vi "Start.vi"(8 "error in (no error)":errorcluster, 11 "TDCManager":T1) -> (0 "error out":errorcluster, 1 "Added time":u64, 2 "Success?":bool=TRUE, 3 "TDCManager":T1)   [LabVIEW 2016, in "HPTDC Driver Library.lvlib"]
uses:
  HPTDC Driver Library.lvlib
  Typedefs/TDCManager.ctl
  C:/Users/CRT Controller/CRTC Labview Application/Source/HPTDC Driver Library Folder/Library files/hptdc_net4_3.7.0_x64.dll
  hptdc_net4_3.7.0_x64.dll
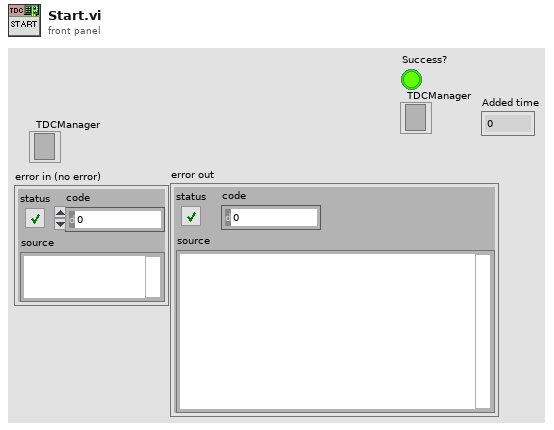
[diagram p1: front panel]
types:
  T1 = typedef "HPTDC Driver Library.lvlib/TDCManager.ctl" = refnum<k24>
  T2 = typedef "Semaphore RefNum" = refnum<k1>
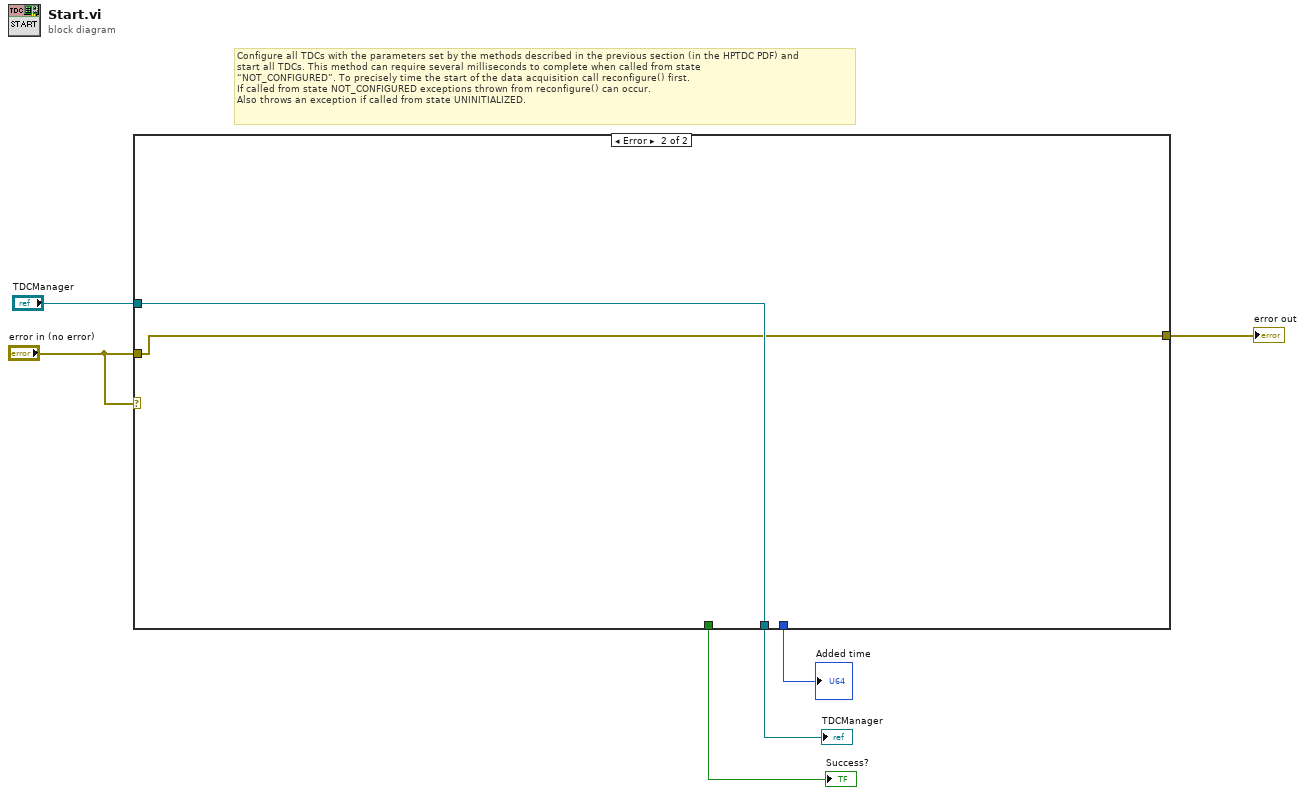
[diagram p0: block diagram]
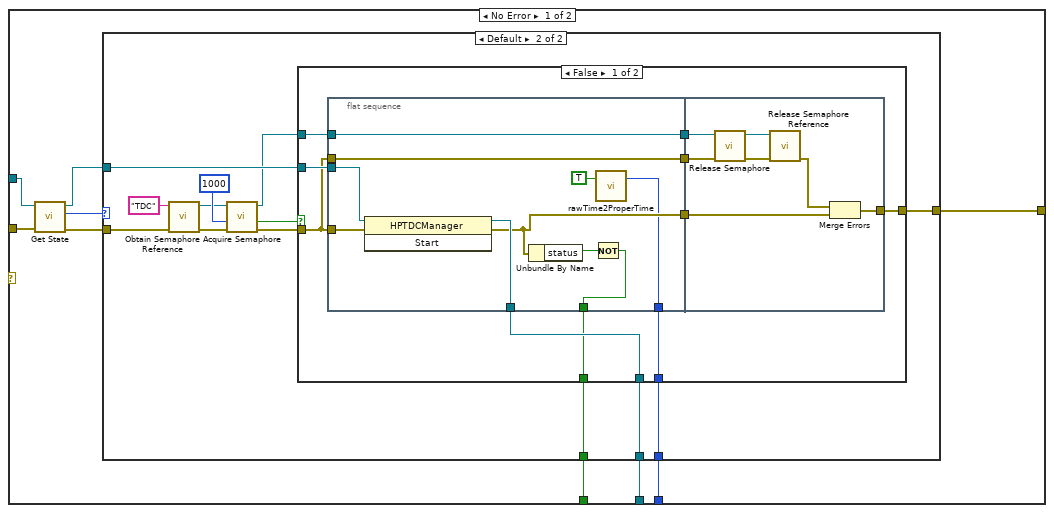
[diagram p2: hidden frame]
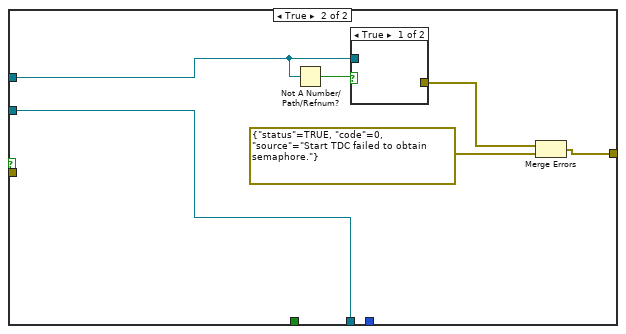
[diagram p4: hidden frame]
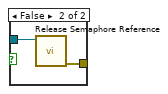
[diagram p5: hidden frame]
diagram:
  # "Configure all TDCs with the parameters set by the methods described in the previous section (in the HPTDC PDF) and\nstart all TDCs. This method can require several milliseconds to complete when called from state\n“NOT_CONFIGURED”. To precisely time the start of the data acquisition call reconfigure() first.\nIf called from state NOT_CONFIGURED exceptions thrown from reconfigure() can occur.\nAlso throws an exception if called from state UNINITIALIZED."
  n1 = case shown="Error" "error in (no error)" {
    tunnel: "TDCManager" -> [w15 w67]
    tunnel: "error in (no error)" -> [w14 w66]
    tunnel: [w10 w66] -> w5
    tunnel: [w9 w67] -> w4
    tunnel: [w8 _] -> w3
    tunnel: [w7 _] -> w2
    frame No Error {
      n2 = call "Get State.vi"("error in"=w14, "TDCManager"=w15) -> ("error out"=w11:errorcluster, "State"=w13:i32, "TDCManager"=w12:T1)  [unwired: 6 in, 1 out]
      n3 = case shown="Default" w13 {
        tunnel: w11 -> [w17 w25]
        tunnel: w12 -> [w16 w30]
        tunnel: [w16 w21] -> w9
        tunnel: [w17 w20] -> w10
        tunnel: [_ w19] -> w8
        tunnel: [_ w18] -> w7
        frame 0 {
        }
        frame Default {
          n4 = call <vilib>:"Obtain Semaphore Reference.vi"("error in (no error)"=w25, "name (unnamed)"="TDC") -> ("error out"=w27:errorcluster, "semaphore"=w28:T2)  [unwired: 3 in, 1 out]
          n5 = call <vilib>:"Acquire Semaphore.vi"("error in (no error)"=w27, "ms timeout (-1)"=1000, "semaphore"=w28) -> ("error out"=w23:errorcluster, "timed out"=w24:bool, "semaphore out"=w22:T2)  [unwired: 2 in]
          n6 = case shown="False" w24 {
            tunnel: w30 -> [w40 w59]
            tunnel: w23 -> [w37 _]
            tunnel: w22 -> [w35 w58]
            tunnel: [w34 w59] -> w21
            tunnel: [w33 w61] -> w20
            tunnel: [w32 _] -> w19
            tunnel: [w31 _] -> w18
            frame False {
              n7 = flat-sequence {
                tunnel: w37 -> [w50]
                tunnel: w40 -> [w49]
                tunnel: [w45] -> w39
                tunnel: w37 -> [w48]
                tunnel: [w48] -> w38
                tunnel: [w47] -> w36
                tunnel: w35 -> [w47]
                tunnel: [w46] -> w34
                tunnel: [w43] -> w32
                tunnel: [w41] -> w31
                tunnel: w39 -> [w57]
                tunnel: w38 -> [w54]
                tunnel: w36 -> [w52]
                tunnel: [w51] -> w33
                frame #0 {
                  n8 = invoke class="HPTDCManager" method="Start"(reference=w49, error in=w50) -> (reference out=w46:T1, error out=w45:errorcluster)  [unwired: 1 in, 1 out]
                  n9 = Unbundle By Name(w45) -> ("status"=w44:bool)
                  n10 = Not(x=w44) -> (.not. x?=w43:bool)
                  n11 = call "rawTime2ProperTime.vi"("Init"=TRUE) -> ("Added time"=w41:u64)  [unwired: 1 in, 1 out]
                }
                frame #1 {
                  n12 = call <vilib>:"Release Semaphore.vi"("error in (no error)"=w54, "semaphore"=w52) -> ("error out"=w55:errorcluster, "semaphore out"=w56:T2)  [unwired: 4 in]
                  n13 = call <vilib>:"Release Semaphore Reference.vi"("error in (no error)"=w55, "semaphore"=w56) -> ("error out"=w53:errorcluster)  [unwired: 8 in, 1 out]
                  n14 = Merge Errors(w53, w57) -> (w51:errorcluster)
                }
              }
            }
            frame True {
              n15 = Not A Number/Path/Refnum?(number/path/refnum=w58) -> (NaN/Path/Refnum?=w63:bool)
              n16 = case shown="True" w63 {
                tunnel: [_ w65] -> w60
                tunnel: w58 -> [_ w64]
                frame True {
                }
                frame False {
                  n17 = call <vilib>:"Release Semaphore Reference.vi"("semaphore"=w64) -> ("error out"=w65:errorcluster)  [unwired: 9 in, 1 out]
                }
              }
              n18 = Merge Errors(w60, errorcluster {"status"=TRUE, "code"=0, "source"="Start TDC failed to obtain semaphore."} ("error out")) -> (w61:errorcluster)
            }
          }
        }
      }
    }
    frame Error {
    }
  }
  "error out" <- w5
  "TDCManager" <- w4
  "Success?" <- w3
  "Added time" <- w2
